vi "_Write XML Configuration.vi"(4 "error in":errorcluster, 7 "Configuration":T1) -> (0 "error out":errorcluster, 3 "XML String":string)   [LabVIEW 2015]
uses:
  Type/_RT Instrument 2.ctl
  Type/_RT Configuration 2.ctl
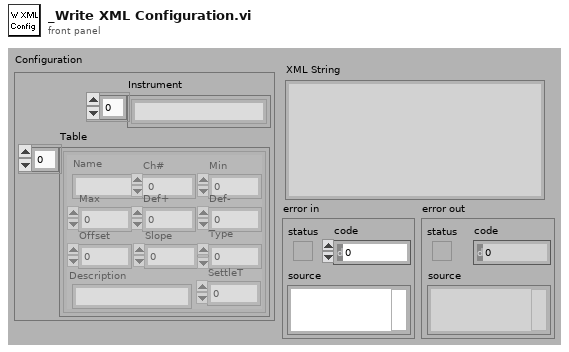
[diagram p1: front panel]
types:
  T1 = typedef "_RT Instrument 2.ctl" = cluster{"Table":T2[], "Instrument":string[]}
  T2 = typedef "_RT Configuration 2.ctl" = cluster{"Name":string, "Ch#":u8, "Min":dbl, "Max":dbl, "Def+":dbl, "Def-":dbl, "Offset":dbl, "Slope":dbl, "Type":u8, "Description":string, "SettleT":dbl}
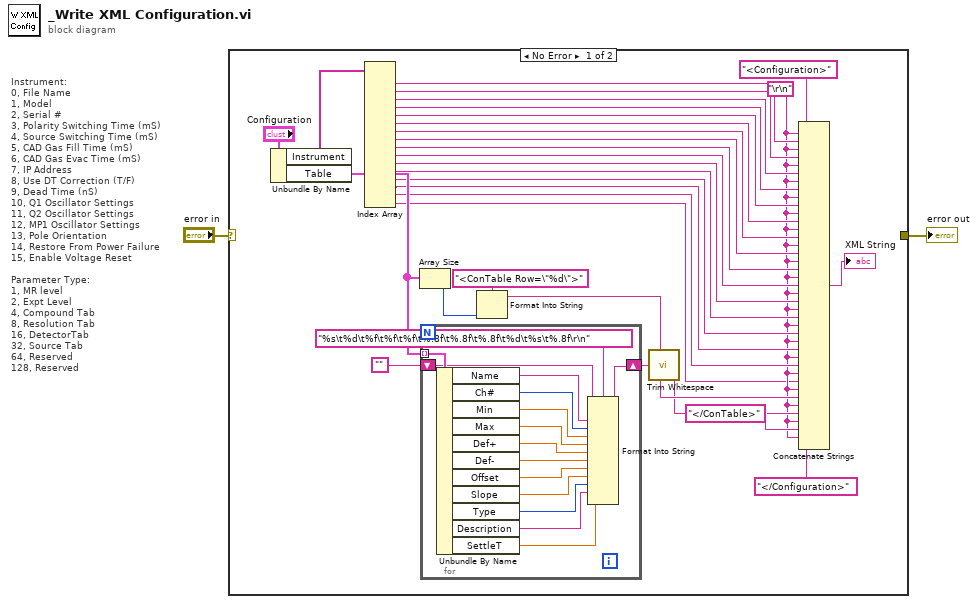
[diagram p0: block diagram]
diagram:
  # "Instrument:\n0, File Name\n1, Model\n2, Serial #\n3, Polarity Switching Time (mS)\n4, Source Switching Time (mS)\n5, CAD Gas Fill Time (mS)\n6, CAD Gas Evac Time (mS)\n7, IP Address\n8, Use DT Correction (T/F)\n9, Dead Time (nS)\n10, Q1 Oscillator Settings\n11, Q2 Oscillator Settings\n12, MP1 Oscillator Settings\n13, Pole Orientation\n14, Restore From Power Failure\n15, Enable Voltage Reset \n\nParameter Type:\n1, MR level\n2, Expt Level\n4, Compound Tab\n8, Resolution Tab\n16, DetectorTab\n32, Source Tab\n64, Reserved\n128, Reserved"
  n1 = case shown="No Error" "error in" {
    selector: "error in" -> [_ w48]
    tunnel: [_ w48] -> w1
    frame No Error {
      w4 = "\r\n"
      n2 = Unbundle By Name("Configuration") -> ("Instrument"=w21:string[], "Table"=w25:T2[])
      n3 = Index Array(array=w21) -> (element #1=w19:string, element #2=w18:string, element #3=w17:string, element #4=w16:string, element #5=w15:string, element #6=w14:string, element #7=w13:string, element #8=w12:string, element #9=w11:string, element #10=w10:string, element #11=w9:string, element #12=w8:string, element #13=w7:string, element #14=w6:string, element #15=w5:string, element #16=w3:string)  [unwired: 16 in]
      n4 = Array Size(array=w25) -> (size(s)=w29:i32)
      n5 = for {
        tunnel: w25 -> [w47] mode=indexing
        shift-right: [w40] -> w23
        shift-left: "" -> [w42]
        n6 = Unbundle By Name(w47) -> ("Name"=w46:string, "Ch#"=w45:u8, "Min"=w44:dbl, "Max"=w37:dbl, "Def+"=w36:dbl, "Def-"=w35:dbl, "Offset"=w34:dbl, "Slope"=w43:dbl, "Type"=w39:u8, "Description"=w38:string, "SettleT"=w33:dbl)
        n7 = Format Into String(format string="%s\t%d\t%f\t%f\t%f\t%.8f\t%.8f\t%.8f\t%d\t%s\t%.8f\r\n", initial string=w42, w46, w45, w44, w37, w36, w35, w34, w43, w39, w38, w33) -> (resulting string=w40:string)  [unwired: 1 in, 1 out]
      }
      n8 = Format Into String(format string="<ConTable Row=\"%d\">", w29) -> (resulting string=w27:string)  [unwired: 2 in, 1 out]
      n9 = call <vilib>:"Trim Whitespace.vi"("string"=w23) -> ("trimmed string"=w22:string)  [unwired: 1 in]
      n10 = Concatenate Strings("<Configuration>" ("format string"), w4, w19, w4, w18, w4, w17, w4, w16, w4, w15, w4, w14, w4, w13, w4, w12, w4, w11, w4, w10, w4, w9, w4, w8, w4, w7, w4, w6, w4, w5, w4, w3, w4, w27, w4, w22, w4, "</ConTable>" ("format string"), w4, "</Configuration>" ("format string")) -> (→"XML String":string)
    }
    frame Error {
    }
  }
  "error out" <- w1
